vi "Controller Write PS Filter Data and Address.vi"(10 "Data":fxp<+/-,20,2>, 11 "Address":u8) -> ()   [LabVIEW 2011, in "Controller VIs.lvlib"]
uses:
  Controller VIs.lvlib
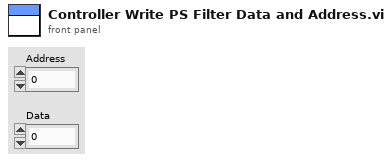
[diagram p1: front panel]
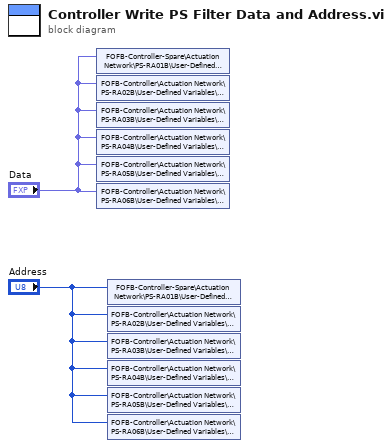
[diagram p0: block diagram]
diagram:
  n1 = shared-variable "FOFB-Controller-Spare\\Actuation Network\\PS-RA01B\\User-Defined Variables\\PS-RA01B-DATA"("Data") -> ()  [unwired: 1 in, 1 out]
  n2 = shared-variable "FOFB-Controller\\Actuation Network\\PS-RA02B\\User-Defined Variables\\PS-RA02B-DATA"("Data") -> ()  [unwired: 1 in, 1 out]
  n3 = shared-variable "FOFB-Controller\\Actuation Network\\PS-RA03B\\User-Defined Variables\\PS-RA03B-DATA"("Data") -> ()  [unwired: 1 in, 1 out]
  n4 = shared-variable "FOFB-Controller\\Actuation Network\\PS-RA04B\\User-Defined Variables\\PS-RA04B-DATA"("Data") -> ()  [unwired: 1 in, 1 out]
  n5 = shared-variable "FOFB-Controller\\Actuation Network\\PS-RA05B\\User-Defined Variables\\PS-RA05B-DATA"("Data") -> ()  [unwired: 1 in, 1 out]
  n6 = shared-variable "FOFB-Controller\\Actuation Network\\PS-RA06B\\User-Defined Variables\\PS-RA06B-DATA"("Data") -> ()  [unwired: 1 in, 1 out]
  n7 = shared-variable "FOFB-Controller-Spare\\Actuation Network\\PS-RA01B\\User-Defined Variables\\PS-RA01B-ADDR"("Address") -> ()  [unwired: 1 in, 1 out]
  n8 = shared-variable "FOFB-Controller\\Actuation Network\\PS-RA02B\\User-Defined Variables\\PS-RA02B-ADDR"("Address") -> ()  [unwired: 1 in, 1 out]
  n9 = shared-variable "FOFB-Controller\\Actuation Network\\PS-RA03B\\User-Defined Variables\\PS-RA03B-ADDR"("Address") -> ()  [unwired: 1 in, 1 out]
  n10 = shared-variable "FOFB-Controller\\Actuation Network\\PS-RA04B\\User-Defined Variables\\PS-RA04B-ADDR"("Address") -> ()  [unwired: 1 in, 1 out]
  n11 = shared-variable "FOFB-Controller\\Actuation Network\\PS-RA05B\\User-Defined Variables\\PS-RA05B-ADDR"("Address") -> ()  [unwired: 1 in, 1 out]
  n12 = shared-variable "FOFB-Controller\\Actuation Network\\PS-RA06B\\User-Defined Variables\\PS-RA06B-ADDR"("Address") -> ()  [unwired: 1 in, 1 out]
